vi "Omni-Bus Inject I16.vi"(6 "Enable":bool, 8 "error in (no error)":errorcluster, 9 "Injected Value":i16, 10 "Tag":string, 11 "Omni_Bus in":refnum<class "Omni_Bus.lvclass">) -> (0 "error out":errorcluster, 3 "Omni_Bus out":refnum<class "Omni_Bus.lvclass">)   [LabVIEW 2021, in "Fault-Injection Bus.lvclass"]
uses:
  Fault-Injection Bus.lvclass
  Omni-Bus/Omni_Bus.lvclass
  Value Type/I16/Fault-Injection_I16.lvclass
  C:/Program Files (x86)/National Instruments/LabVIEW 2021/vi.lib/TSA/Abstract Data Classes/Abs_Types/Type/Abs_Type.lvclass
  <vilib>/TSA/Abstract Data Classes/Abs_Types/Type/Abs_Type.lvclass/Abs_Type.ctl
  Omni-Bus/Omni_Bus.lvclass/Omni_Bus.ctl
  <vilib>/Utility/error.llb/Clear Errors.vi
  Omni-Bus/Properties/Read Var Map.vi
  <vilib>/TSA/Abstract Data Classes/Abs_Types/Type/Properties/Read Tag.vi
  <vilib>/TSA/Abstract Data Classes/Abs_Types/Value/Abs_Value.lvclass
  Omni-Bus/Support/Check For Read Only Error.vi
  Omni-Bus/Support/Incorrect Tag String Error.vi
  <vilib>/TSA/Abstract Data Classes/Abs_Types/Type/Abs_Type.lvclass
  Fault-Injection Bus.lvclass/Fault-Injection Bus.ctl
  C:/Program Files (x86)/National Instruments/LabVIEW 2021/vi.lib/TSA/Abstract Data Classes/Abs_Types/I16 Integer/Abs_I16 Integer.lvclass
  C:/Program Files (x86)/National Instruments/LabVIEW 2021/vi.lib/TSA/Abstract Data Classes/Abs_Types/Integer/Abs_Integer.lvclass
  C:/Program Files (x86)/National Instruments/LabVIEW 2021/vi.lib/TSA/Abstract Data Classes/Abs_Types/Numeric/Abs_Numeric.lvclass
  C:/Program Files (x86)/National Instruments/LabVIEW 2021/vi.lib/TSA/Abstract Data Classes/Abs_Types/Value/Abs_Value.lvclass
  C:/TSA/Omni-Bus/Source/Fault-Injection Bus/Support/Interfaces/I16/Fault-Injection_I16_Type.lvclass
  C:/TSA/Omni-Bus/Source/Fault-Injection Bus/Support/Interfaces/Type/Fault-Injection_Type.lvclass
  C:/TSA/Omni-Bus/Source/Fault-Injection Bus/Support/Value Type/I16/Fault-Injection_I16.lvclass
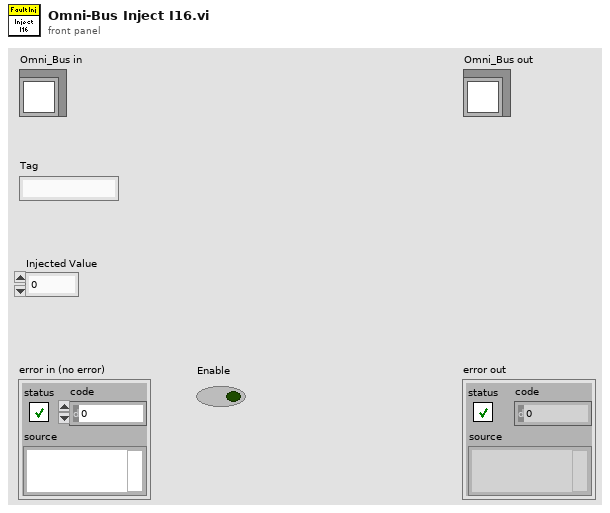
[diagram p1: front panel]
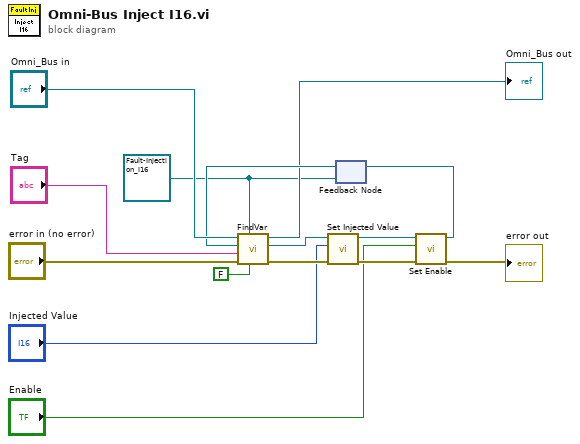
[diagram p0: block diagram]
diagram:
  w1 = refnum<class "Fault-Injection_I16.lvclass"> refnum ("Fault-Injection_Boolean out")
  n1 = feedback #1(w1) -> (w11:refnum<class "Fault-Injection_I16.lvclass">)
  n2 = call "FindVar.vi"("Write?"=FALSE, "Abs_Type"=w1, "error in (no error)"="error in (no error)", "Tag"="Tag", "Abs_Type Default"=w11, "Var Bus in"="Omni_Bus in") -> ("error out"=w14:errorcluster, "Abs_Type Found"=w13:refnum<class "Fault-Injection_I16.lvclass">, "Var Bus out"=→"Omni_Bus out":refnum<class "Omni_Bus.lvclass">)  [unwired: 2 in, 1 out]
  n3 = call-dynamic "Set Injected Value.vi"("error in (no error)"=w14, "Value"="Injected Value", "Fault-Injection_Boolean in"=w13) -> ("error out"=w10:errorcluster, "Fault-Injection_Boolean out"=w9:refnum<class "Fault-Injection_I16.lvclass">)  [unwired: 7 in]
  n4 = call-dynamic "Set Enable.vi"("error in (no error)"=w10, "Enable"="Enable", "Fault-Injection_Boolean in"=w9) -> ("error out"=→"error out":errorcluster, "Fault-Injection_Boolean out"=w8:refnum<class "Fault-Injection_I16.lvclass">)  [unwired: 7 in]
  n5 = feedback-in #1(w8) -> ()
